vi "TDC_getHistogrami.vi"(0 "Channel A":i32, 5 "Channel B":i32, 7 "Reset":bool, 9 "Histogram Size":i32, 11 "Error In":errorcluster) -> (2 "Events B":i32, 3 "Events A":i32, 4 "Data Count":i32, 6 "TooSmall":i32, 8 "TooLarge":i32, 10 "Data":i32[](array[numeric]), 13 "Exposure Time":i64, 15 "Error Out":errorcluster)   [LabVIEW 2013]
uses:
  QUTAU-15_06_25/userlib/lib/tdcbase.dll
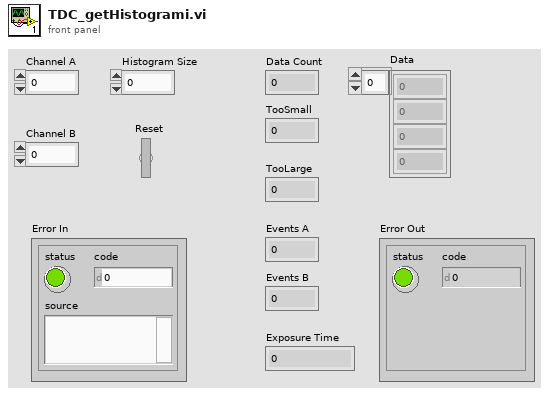
[diagram p1: front panel]
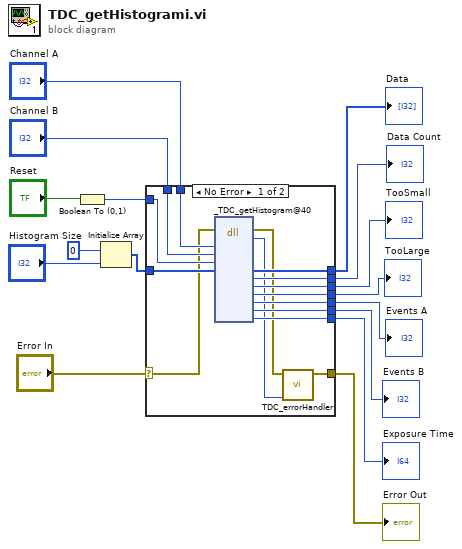
[diagram p0: block diagram]
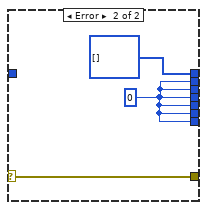
[diagram p2: hidden frame]
diagram:
  n1 = Boolean To (0,1)(Boolean="Reset") -> (0, 1=w9:i16)
  n2 = Initialize Array(0, "Histogram Size") -> (w11:i32[])
  n3 = case shown="No Error" "Error In" {
    selector: "Error In" -> [w20 w34]
    tunnel: [w17 w34] -> w15
    tunnel: [w31 i32[] []] -> w14
    tunnel: w11 -> [w30 _]
    tunnel: w9 -> [w29 _]
    tunnel: [w28 w32] -> w8
    tunnel: "Channel B" -> [w27 _]
    tunnel: "Channel A" -> [w26 _]
    tunnel: [w25 w32] -> w5
    tunnel: [w24 w32] -> w4
    tunnel: [w23 w32] -> w3
    tunnel: [w22 w32] -> w2
    tunnel: [w21 w32] -> w1
    frame No Error {
      n4 = dll-call lib="C:/Users/science/Desktop/NVExperimeent/Labview/QUTAU-15_06_25/userlib/lib/tdcbase.dll" fn="_TDC_getHistogram@40"(error in=w20, "chanA"=w26, "chanB"=w27, "reset"=w29, "data"=w30) -> (error out=w19:errorcluster, "return type"=w18:i32, "data"=w31:i32[], "count"=w28:i32, "tooSmall"=w25:i32, "tooLarge"=w24:i32, "eventsA"=w23:i32, "eventsB"=w22:i32, "expTime"=w21:i64)  [unwired: 11 in, 1 out]
      n5 = call "TDC_errorHandler.vi"("quTAU Return Code"=w18, "Error In"=w19) -> ("Error Out"=w17:errorcluster)  [unwired: 9 in]
    }
    frame Error {
      w32 = 0
    }
  }
  "Error Out" <- w15
  "Data" <- w14
  "Data Count" <- w8
  "TooSmall" <- w5
  "TooLarge" <- w4
  "Events A" <- w3
  "Events B" <- w2
  "Exposure Time" <- w1
